vi "OE2011&OE2021_Configure Oscillator Reference.vi"(7 "OE2011&OE2021_\nConfigure Osc Ref":T1={"Oscillator Source"=0, "Oscillator Frequency(Hz)"=1000.0, "Oscillator Channel"=1, "External Ref Slope"=0, "Instrument Mode "=10, "Oscillator Mode"=0} {"Oscillator Mode" items=["External", "Internal"]; "Instrument Mode" items=["OE2011"=10, "OE2021"=11]; "External Ref Slope" items=["TTL Rising Edge", "TTL Fallling Edge", "Sine Zero Crossing"]; "Oscillator Channel" items=["OSC1"=1, "OSC2"=2]; "Oscillator Frequency(Hz)" min=0.001 max=1500000.0 format="%#.3f"; "Oscillator Source" items=["Ref In", "Signal In", "Aux In 1", "Aux In 2", "Aux In 3", "Aux In 4", "Trig In"]}, 8 "Error in (no error)":errorcluster caption="error out（no error）", 9 "Remote Mode":u16(ring)=1 items=["USB", "RS232", "GPIB", "Ethernet"], 10 "Connection ID in":refnum<k5>, 11 "VISA resource name":refnum<visa-resource-name>) -> (0 "Error out":errorcluster caption="error out", 1 "Output String":string, 2 "Connection ID out":refnum<k5>, 3 "VISA resource  out":refnum<visa-resource-name>)   [LabVIEW 2011]
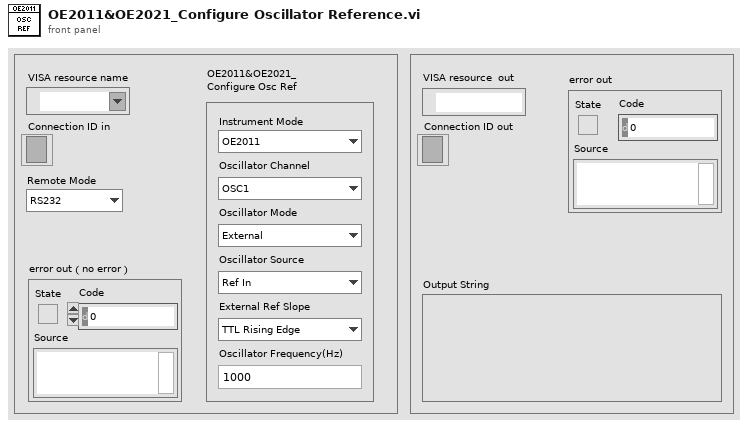
[diagram p1: front panel]
types:
  T1 = cluster{"Oscillator Source":u16, "Oscillator Frequency(Hz)":dbl, "Oscillator Channel":u8, "External Ref Slope":u16, "Instrument Mode ":u16, "Oscillator Mode":u16}
  T2 = enum16{"ISRC", "IGND", "ICPL", "ILIN", "PHAS", "FMOD", "RSLP", "FREQ", "SWPT", "SLLM", "SULM", "SSLL", "SSLG", "STLM", "SWRM", "IRNG", "SENS", "RMOD", "OFLT", "OFSL", "SYNC", "DMOD", "HARM", "DARB", "SWVT", "SLVL", "SVLL", "SVUL", "SVSL", "SVSG", "SVTM", "SVRM", "RALL", "SNAP", "OUTP", "OAUX", "COUT", "CAUX", "COFP", "CEXP", "FPOP", "OEXP", "*IDN", "*RST", "OVLD", "INOV", "GNOV", "*PLL", "SSET", "RSET", "AGAN", "APHS", "ARSV", "ASCL", "EQCD", "EQCS", "SPED", "SRAT", "SLEN", "SSLE", "STRG", "SPRM", "STRD", "PAUS", "REST", "SPTS", "TRCA", "TEMP", "RSTU", "IHNZ", "DEQU", "SADD", "ARNG", "CSPE", "ISRCD", "IGNDD", "ICPLD", "ILIND", "PHASD", "FMODD", "RSLPD", "FREQD", "SWPTD", "SLLMD", "SULMD", "SSLLD", "SSLGD", "STLMD", "SWRMD", "SENSD", "RMODD", "OFLTD", "OFSLD", "SYNCD", "HARMD", "EQCDD", "EQCSD", "SNAPD", "OUTPD", "SWVTD", "SLVLD", "SVLLD", "SVULD", "SVSLD", "SVSGD", "SVTMD", "SVRMD", "SVDCD", "ARSVD", "AGAND", "APHSD", "ASCLD", "FPOPD", "CAUXD", "OEXPD", "SPEDD", "SRATD", "SLEND", "SSLED", "STRGD", "SPRMD", "STRDD", "PAUSD", "RESTD", "SPTSD", "TRCAD", "*IDND", "*RSTD", "INOVD", "GNOVD", "*PLLD", "SSETD", "RSETD", "RALLD"}
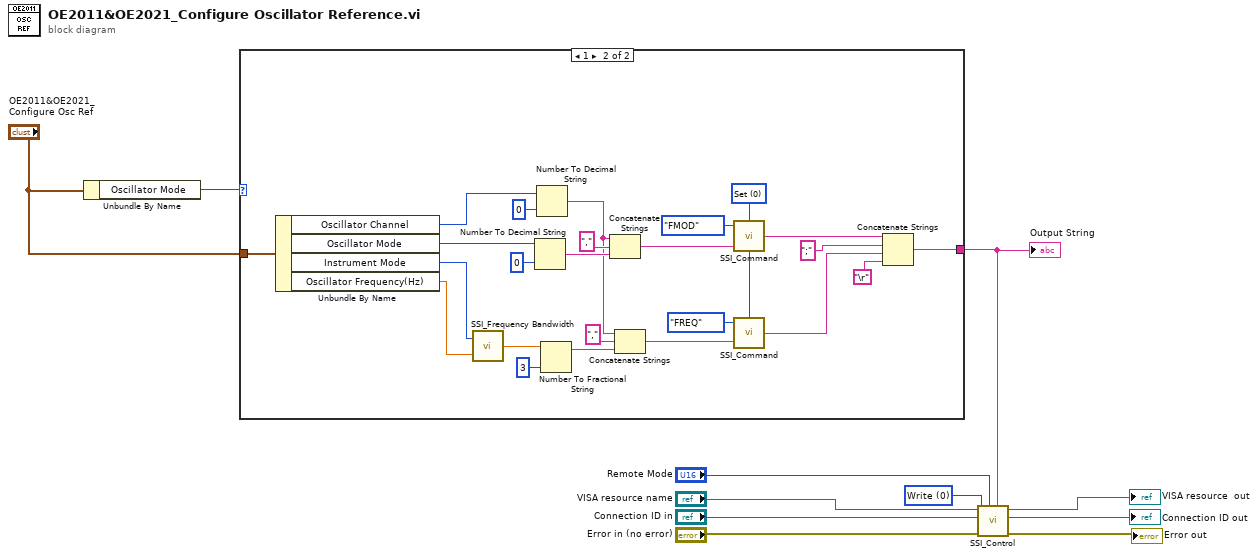
[diagram p0: block diagram]
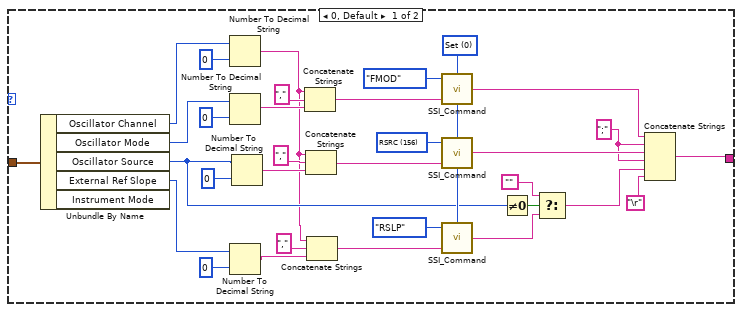
[diagram p2: hidden frame]
diagram:
  w9 = u16 0 items=["Write", "Read"] ("Control")
  n1 = Unbundle By Name("OE2011&OE2021_\nConfigure Osc Ref") -> ("Oscillator Mode"=w4:u16)
  n2 = case shown="1" w4 {
    tunnel: "OE2011&OE2021_\nConfigure Osc Ref" -> [w41 w65]
    tunnel: [w40 w64] -> w5
    frame 0, Default {
      w29 = u16 156 items=["ISRC", "IGND", "ICPL", "ILIN", "PHAS", "FMOD", "RSLP", "FREQ", "SWPT", "SLLM", "SULM", "SSLL", "SSLG", "STLM", "SWRM", "IRNG", "SENS", "RMOD", "OFLT", "OFSL", "SYNC", "DMOD", "HARM", "DARB", "SWVT", "SLVL", "SVLL", "SVUL", "SVSL", "SVSG", "SVTM", "SVRM", "RALL", "SNAP", "OUTP", "OAUX", "COUT", "CAUX", "COFP", "CEXP", "FPOP", "OEXP", "*IDN", "*RST", "OVLD", "INOV", "GNOV", "*PLL", "SSET", "RSET", "AGAN", "APHS", "ARSV", "ASCL", "EQCD", "EQCS", "SPED", "SRAT", "SLEN", "SSLE", "STRG", "SPRM", "STRD", "PAUS", "REST", "SPTS", "TRCA", "TEMP", "RSTU", "INHZ", "DEQU", "SADD", "ARNG", "CSPE", "ISRCD", "IGNDD", "ICPLD", "ILIND", "PHASD", "FMODD", "RSLPD", "FREQD", "SWPTD", "SLLMD", "SULMD", "SSLLD", "SSLGD", "STLMD", "SWRMD", "SENSD", "RMODD", "OFLTD", "OFSLD", "SYNCD", "HARMD", "EQCDD", "EQCSD", "SNAPD", "OUTPD", "SWVTD", "SLVLD", "SVLLD", "SVULD", "SVSLD", "SVSGD", "SVTMD", "SVRMD", "SVDCD", "ARSVD", "AGAND", "APHSD", "ASCLD", "FPOPD", "CAUXD", "OEXPD", "SPEDD", "SRATD", "SLEND", "SSLED", "STRGD", "SPRMD", "STRDD", "PAUSD", "RESTD", "SPTSD", "TRCAD", "*IDND", "*RSTD", "INOVD", "GNOVD", "*PLLD", "SSETD", "RSETD", "RALLD", "NIPA", "NSMA", "NGWA", "NMAC", "NMOD", "TRIG", "TRCB", "INHZD", "ISAMD", "IRAGD", "RRAGD", "SOFFD", "DMODD", "COUTD", "COFPD", "CEXPD", "ARNGD", "OAUXD", "TRIM", "SUITD", "SNHZD", "AOFSD", "RSRC", "FEXT", "FINT", "DSRC"] ("Command Type")
      w30 = u16 0 items=["Set", "Query"] ("Opera")
      w21 = ";" ("替换字符串(\"\")")
      n3 = Unbundle By Name(w41) -> ("Oscillator Channel"=w34:u8, "Oscillator Mode"=w33:u16, "Oscillator Source"=w26:u16, "External Ref Slope"=w28:u16)  [unwired: 1 out]
      n4 = Number To Decimal String(number=w34, width (-)=i16 0 ("精度(6)")) -> (decimal integer string=w12:string)
      n5 = Number To Decimal String(number=w33, width (-)=i16 0 ("精度(6)")) -> (decimal integer string=w35:string)
      n6 = Number To Decimal String(number=w28, width (-)=i16 0 ("精度(6)")) -> (decimal integer string=w16:string)
      n7 = Number To Decimal String(number=w26, width (-)=i16 0 ("精度(6)")) -> (decimal integer string=w25:string)
      n8 = Concatenate Strings(w12, "," ("字符串"), w35) -> (w32:string)
      n9 = Concatenate Strings(w12, "," ("字符串"), w25) -> (w24:string)
      n10 = Concatenate Strings(w12, "," ("字符串"), w16) -> (w15:string)
      n11 = call "SSI_Command.vi"("Opera"=w30, "Paramter"=w32, "Command Type"=T2."FMOD") -> ("Output string"=w23:string)  [unwired: 1 in]
      n12 = call "SSI_Command.vi"("Opera"=w30, "Paramter"=w24, "Command Type"=w29) -> ("Output string"=w22:string)  [unwired: 1 in]
      n13 = call "SSI_Command.vi"("Opera"=w30, "Paramter"=w15, "Command Type"=T2."RSLP") -> ("Output string"=w20:string)  [unwired: 1 in]
      n14 = Not Equal To 0?(x=w26) -> (x != 0?=w31:bool)
      n15 = Select(t="", s=w31, f=w20) -> (s? t:f=w14:string)
      n16 = Concatenate Strings(w23, w21, w22, w21, w14, "\r") -> (w40:string)
    }
    frame 1 {
      w66 = u16 0 items=["Set", "Query"] ("Opera")
      n17 = Unbundle By Name(w65) -> ("Oscillator Channel"=w57:u8, "Oscillator Mode"=w53:u16, "Instrument Mode"=w51:u16, "Oscillator Frequency(Hz)"=w52:dbl)
      n18 = call "SSI_Frequency Bandwidth.vi"("Frequency"=w52, "Instrument Mode"=w51) -> ("Output"=w60:dbl)  [unwired: 1 in]
      n19 = Number To Decimal String(number=w53, width (-)=i16 0 ("精度(6)")) -> (decimal integer string=w54:string)
      n20 = Number To Decimal String(number=w57, width (-)=i16 0 ("精度(6)")) -> (decimal integer string=w49:string)
      n21 = Number To Fractional String(number=w60, precision (6)=i16 3 ("精度(6)")) -> (F-format string=w50:string)  [unwired: 2 in]
      n22 = Concatenate Strings(w49, "," ("字符串"), w54) -> (w56:string)
      n23 = Concatenate Strings(w49, "," ("字符串"), w50) -> (w47:string)
      n24 = call "SSI_Command.vi"("Opera"=w66, "Paramter"=w56, "Command Type"=T2."FMOD") -> ("Output string"=w46:string)  [unwired: 1 in]
      n25 = call "SSI_Command.vi"("Opera"=w66, "Paramter"=w47, "Command Type"=T2."FREQ") -> ("Output string"=w44:string)  [unwired: 1 in]
      n26 = Concatenate Strings(w46, ";", w44, "\r") -> (w64:string)
    }
  }
  "Output String" <- w5
  n27 = call "SSI_Control.vi"("Write Buffer"=w5, "Remote Mode"="Remote Mode", "Error in (no error)"="Error in (no error)", "Control"=w9, "Connection ID in"="Connection ID in", "VISA resource name"="VISA resource name") -> ("Error out"=→"Error out":errorcluster, "Connection ID out"=→"Connection ID out":refnum<k5>, "VISA resource  out"=→"VISA resource  out":refnum<visa-resource-name>)  [unwired: 2 in, 1 out]
